vi "Send Character.vi"(8 "error in":errorcluster, 10 "Character to send":string) -> (0 "error out":errorcluster)   [LabVIEW 2025, in "Keyboard.lvlib"]
doc: "Broadcast the supplied character to any listening module or VI.\n\n_____\nCreated using DQMH Framework: Event Scripter 7.1.0.1503."
uses:
  Keyboard.lvlib
  Send Character Argument--cluster.ctl
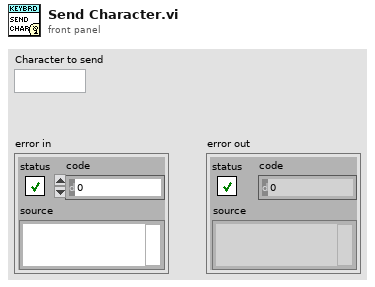
[diagram p1: front panel]
types:
  T1 = typedef "Keyboard.lvlib/Send Character Argument--cluster.ctl" = cluster{"Character to send":string}
  T2 = typedef "Keyboard.lvlib/Broadcast Events--cluster.ctl" = cluster{"Module Did Init":refnum<user-event>, "Status Updated":refnum<user-event>, "Error Reported":refnum<user-event>, "Module Did Stop":refnum<user-event>, "Update Module Execution Status":refnum<user-event>, "Send Character":refnum<user-event>}
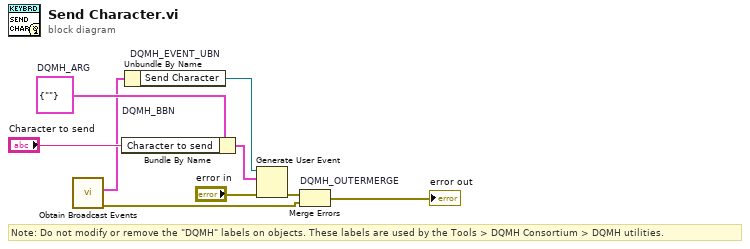
[diagram p0: block diagram]
diagram:
  w4 = T1 {"Character to send"=""}  # DQMH_ARG
  # "Note: Do not modify or remove the \"DQMH\" labels on objects. These labels are used by the Tools > DQMH Consortium > DQMH utilities."
  n1 = call "Obtain Broadcast Events.vi"() -> ("error out"=w2:errorcluster, "Keyboard Broadcast Events"=w1:T2)  [unwired: 10 in]
  n2 = Bundle By Name "DQMH_BBN"(cluster=w4, "Character to send"="Character to send") -> (w7:T1)
  n3 = Unbundle By Name "DQMH_EVENT_UBN"(w1) -> ("Send Character"=w6:refnum<user-event>)
  n4 = Generate User Event(user event=w6, event data cluster=w7, error in="error in") -> (error out=w5:errorcluster)  [unwired: 1 in, 1 out]
  n5 = Merge Errors "DQMH_OUTERMERGE"(w5, w2) -> (→"error out":errorcluster)
